vi "Refresh GUI.vi"(8 "error in (no error)":errorcluster, 11 "PluginGUI in":refnum<class "PluginGUI.lvclass">) -> (0 "error out":errorcluster, 3 "PluginGUI out":refnum<class "PluginGUI.lvclass">)   [LabVIEW 2020, in "VolatusGUI.lvlib" / "PluginGUI.lvclass"]
uses:
  PluginGUI.lvclass
  PluginGUI.lvclass/PluginGUI.ctl
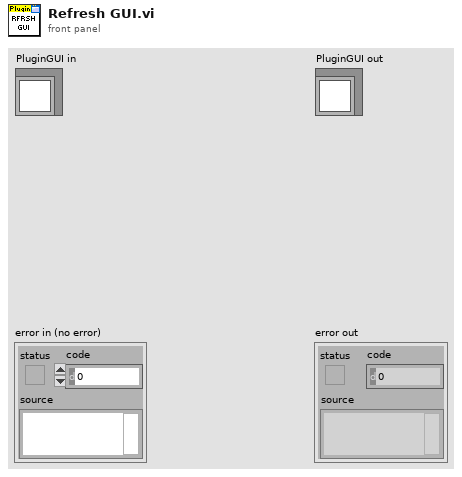
[diagram p1: front panel]
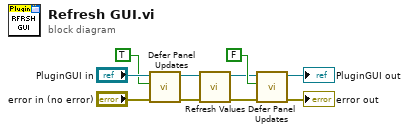
[diagram p0: block diagram]
diagram:
  n1 = call "Defer Panel Updates.vi"("error in (no error)"="error in (no error)", "Defer Panel Updates"=TRUE, "PluginGUI in"="PluginGUI in") -> ("error out"=w9:errorcluster, "PluginGUI out"=w2:refnum<class "PluginGUI.lvclass">)  [unwired: 7 in]
  n2 = call "Refresh Values.vi"("error in (no error)"=w9, "PluginGUI in"=w2) -> ("error out"=w3:errorcluster, "PluginGUI out"=w1:refnum<class "PluginGUI.lvclass">)  [unwired: 8 in]
  n3 = call "Defer Panel Updates.vi"("error in (no error)"=w3, "Defer Panel Updates"=FALSE, "PluginGUI in"=w1) -> ("error out"=→"error out":errorcluster, "PluginGUI out"=→"PluginGUI out":refnum<class "PluginGUI.lvclass">)  [unwired: 7 in]
